vi "FiberSpectrograph_getSample_loopTimems.vi"(8 "error in (no error)":errorcluster, 11 "loopTime_ms_Ctl":T1) -> (0 "error out":errorcluster, 2 "function return":i32, 3 "loopTime_ms_Ctl out":T1)   [LabVIEW 2016, in "SALLV_FiberSpectrograph.lvlib"]
doc: "int FiberSpectrograph_shm_getSample_loopTime_msLV(FiberSpectrograph_loopTime_msLV *loopTime_ms_Ctl );"
uses:
  SALLV_FiberSpectrograph.lvlib
  DataTypes/loopTime_ms.ctl
  SALLV_FiberSpectrograph.so
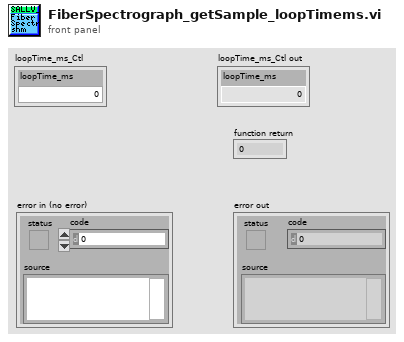
[diagram p1: front panel]
types:
  T1 = typedef "SALLV_FiberSpectrograph.lvlib/loopTime_ms.ctl" = cluster{"loopTime_ms":dbl}
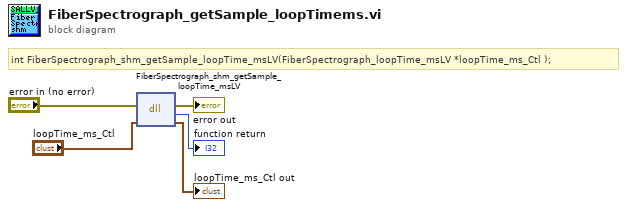
[diagram p0: block diagram]
diagram:
  # "int FiberSpectrograph_shm_getSample_loopTime_msLV(FiberSpectrograph_loopTime_msLV *loopTime_ms_Ctl );"
  n1 = dll-call lib="home/harini/tcs/sallv_FiberSpectrometer/SALLV_FiberSpectrograph.*" fn="FiberSpectrograph_shm_getSample_loopTime_msLV"(error in="error in (no error)", "loopTime_ms_Ctl"="loopTime_ms_Ctl") -> (error out=→"error out":errorcluster, →"function return":i32, "loopTime_ms_Ctl"=→"loopTime_ms_Ctl out":T1)  [unwired: 2 in, 1 out]
